vi "Copy File with Ask.vi"(6 "Use Prev Answer":bool, 8 "Error In":errorcluster, 9 "On File Coillision":T1={"Dest is Newer & RO"=enum."Skip", "Dest is Newer & RW"=enum."Skip", "Dest is Older & RO"=enum."Ask", "Dest is Older & RW"=enum."Overwrite Siliently"}, 10 "Destination Folder":path, 11 "Source File":path) -> (0 "Error Out":errorcluster, 3 "New Path":path, 4 "Use same answer for all":bool)   [LabVIEW 2018]
doc: "Recursively copies files from one folder to another.\nOptions for file collisions:\n Throw Error\n Ask\n Ask if Source is Older\n Overwrite Silently"
uses:
  File Collision Options.ctl
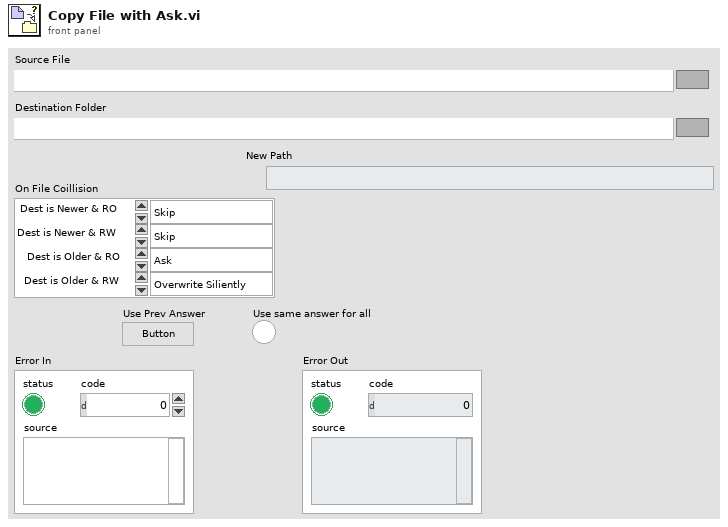
[diagram p1: front panel]
types:
  T1 = typedef "File Collision Options.ctl" = cluster{"Dest is Newer & RO":enum16{"Throw Error", "Ask", "Skip", "Overwrite Siliently"}, "Dest is Newer & RW":enum16{"Throw Error", "Ask", "Skip", "Overwrite Siliently"}, "Dest is Older & RO":enum16{"Throw Error", "Ask", "Skip", "Overwrite Siliently"}, "Dest is Older & RW":enum16{"Throw Error", "Ask", "Skip", "Overwrite Siliently"}}
  T2 = typedef "Dialog Buttons.ctl" = enum32{"No Selection", "Copy", "Skip Ahead", "Stop"}
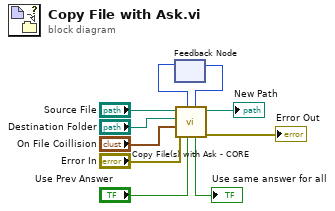
[diagram p0: block diagram]
diagram:
  n1 = feedback #1() -> (w4:T2)  [unwired: 1 in]
  n2 = call "Copy File(s) with Ask - CORE.vi"("Use Prev Answer"="Use Prev Answer", "Prev Answer"=w4, "Error In"="Error In", "On File Coillision"="On File Coillision", "Destination Foilder"="Destination Folder", "Source File"="Source File") -> ("Error Out"=→"Error Out":errorcluster, "New Path"=→"New Path":path, "Use same answer for all"=→"Use same answer for all":bool, "Answer"=w3:T2)  [unwired: 2 in]
  n3 = feedback-in #1(w3) -> ()
